vi "读开关配置文件.vi"(7 "Switch path":path=path "G:/2023项目/陆译电子/0008 User Management/Config/Switch.ini", 10 "型号":string="SP3T") -> (2 "Value":T1)   [LabVIEW 2020]
uses:
  <vilib>/Utility/config.llb/Read Key (String).vi
  <vilib>/Utility/config.llb/NI_LVConfig.lvlib
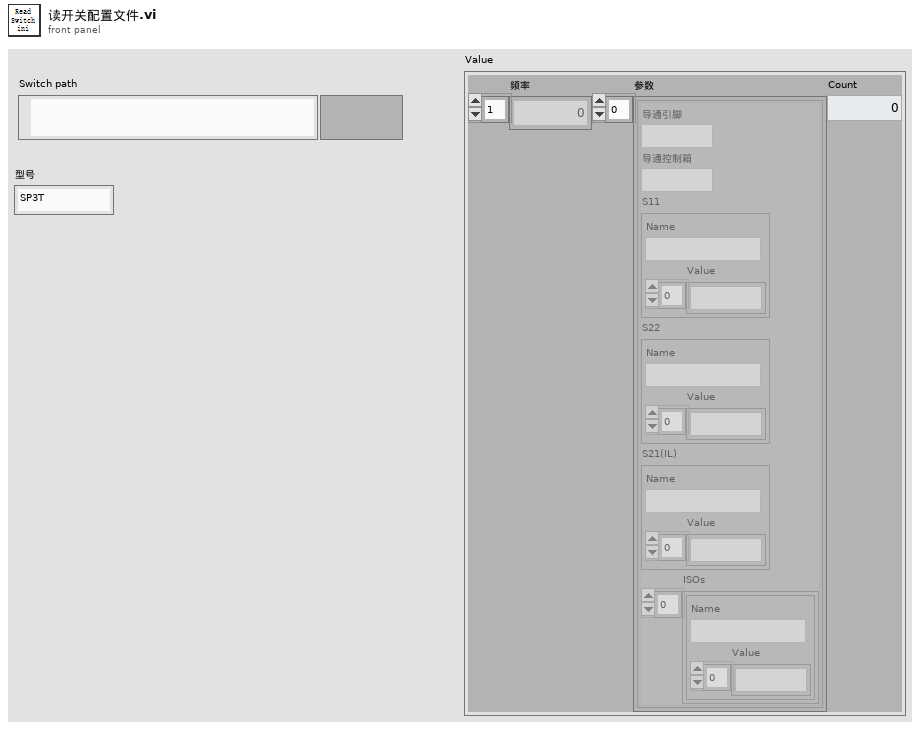
[diagram p1: front panel]
types:
  T1 = cluster{"频率":dbl[], "参数 ":cluster{"导通引脚":string, "导通控制箱":string, "S11":cluster{"Name":string, "Value":string[]}, "S22":cluster{"Name":string, "Value":string[]}, "S21(IL)":cluster{"Name":string, "Value":string[]}, "ISOs":cluster{"Name":string, "Value":string[]}[]}[], "Count":i32}
  T2 = typedef "NI_LVConfig.lvlib/Config Data RefNum.ctl" = refnum<k1>
  T3 = cluster{"导通引脚":string, "导通控制箱":string, "S11":cluster{"Name":string, "Value":string[]}, "S22":cluster{"Name":string, "Value":string[]}, "S21(IL)":cluster{"Name":string, "Value":string[]}, "ISOs":cluster{"Name":string, "Value":string[]}[]}
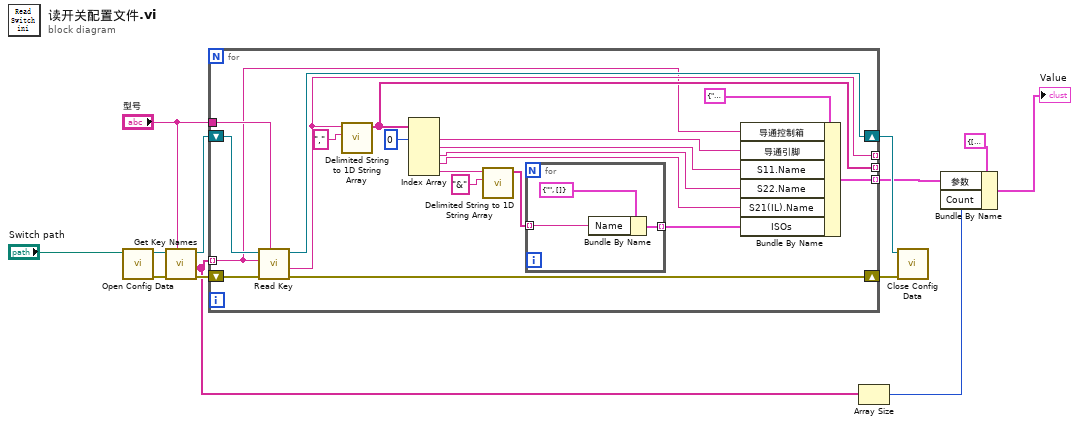
[diagram p0: block diagram]
diagram:
  n1 = call <vilib>:"Open Config Data.vi"("configuration file path"="Switch path") -> ("error out"=w11:errorcluster, "refnum"=w12:T2)  [unwired: 8 in, 1 out]
  n2 = call <vilib>:"Get Key Names.vi"("section"="型号", "error in (no error)"=w11, "refnum"=w12) -> ("error out"=w8:errorcluster, "key names"=w3:string[], "refnum out"=w10:T2)  [unwired: 5 in, 1 out]
  n3 = for {
    tunnel: "型号" -> [w29]
    shift-right: [w32] -> w9
    shift-left: w10 -> [w33]
    shift-right: [w30] -> w7
    shift-left: w8 -> [w31]
    tunnel: w3 -> [w25] mode=indexing
    tunnel: [w28] -> _ mode=indexing
    tunnel: [w26] -> _ mode=indexing
    tunnel: [w23] -> w5 mode=indexing
    n4 = call-poly <vilib>:"Read Key.vi"("section"=w29, "error in (no error)"=w31, "key"=w25, "refnum"=w33) -> ("error out"=w30:errorcluster, "value"=w28:string, "refnum out"=w32:T2)  [unwired: 4 in, 1 out]
    n5 = call <vilib>:"Delimited String to 1D String Array.vi"("delimiter"=",", "delimited string"=w28) -> ("string array"=w26:string[])  [unwired: 9 in]
    n6 = Index Array(array=w26, index #1=0 ("index")) -> (element #1=w24:string, element #2=w20:string, element #3=w19:string, element #4=w18:string, element #5=w17:string)  [unwired: 4 in]
    n7 = call <vilib>:"Delimited String to 1D String Array.vi"("delimiter"="&", "delimited string"=w17) -> ("string array"=w15:string[])  [unwired: 9 in]
    n8 = for {
      tunnel: w15 -> [w35] mode=indexing
      tunnel: [w34] -> w14 mode=indexing
      n9 = Bundle By Name(cluster=cluster{"Name":string, "Value":string[]} {"Name"="", "Value"=[]} ("S21(ISO)"), "Name"=w35) -> (w34:cluster{"Name":string, "Value":string[]})
    }
    n10 = Bundle By Name(cluster=T3 {"导通引脚"="", "导通控制箱"="", "S11"={"Name"="", "Value"=[]}, "S22"={"Name"="", "Value"=[]}, "S21(IL)"={"Name"="", "Value"=[]}, "ISOs"=[]} ("Cluster 2"), "导通控制箱"=w25, "导通引脚"=w24, "S11.Name"=w20, "S22.Name"=w19, "S21(IL).Name"=w18, "ISOs"=w14) -> (w23:T3)
  }
  n11 = Array Size(array=w3) -> (size(s)=w2:i32)
  n12 = call <vilib>:"Close Config Data.vi"("error in (no error)"=w7, "refnum"=w9) -> ()  [unwired: 8 in, 2 out]
  n13 = Bundle By Name(cluster=T1 {"频率"=[], "参数 "=[], "Count"=0} ("Value"), "参数"=w5, "Count"=w2) -> (→"Value":T1)
